vi "oa_Analog Tacho Hysteresis(1 Channel).vi"(0 "input signal":dbl[](array[numeric]), 1 "reset? (T)":bool=TRUE, 5 "threshold (auto)":dbl=inf format="%.2f", 7 "slope (Rising)":u16(ring) items=["Rising", "Falling"], 9 "hysteresis(0)":dbl format="%.2f", 11 "error in (no error)":errorcluster) -> (4 "output signal":dbl[](array[numeric]), 15 "error out":errorcluster)   [LabVIEW 2017, in "SoundVib_TachProcess.lvlib"]
doc: "This VI works like a hysteresis comparater. It can transform the input tachometer signal into a standard square waveform, ignoring small pulsed caused by harmonics or noise. By setting the hystersis value properly, it can make the speed tracking more accurately."
uses:
  <vilib>/addons/Sound and Vibration/Order Analysis/Tach Process/SoundVib_TachProcess.lvlib
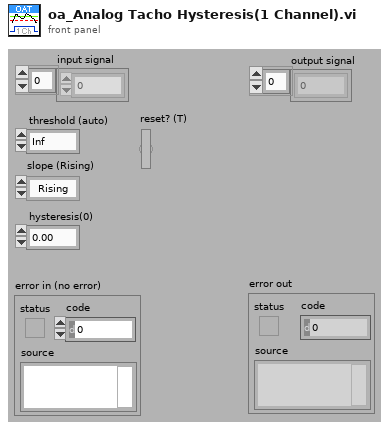
[diagram p1: front panel]
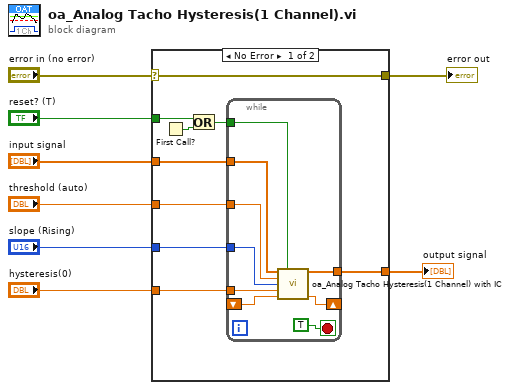
[diagram p0: block diagram]
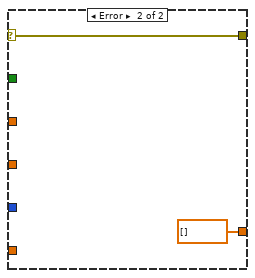
[diagram p2: hidden frame]
diagram:
  n1 = case shown="No Error" "error in (no error)" {
    selector: "error in (no error)" -> [w15 w28]
    tunnel: "reset? (T)" -> [w16 _]
    tunnel: "hysteresis(0)" -> [w10 _]
    tunnel: "threshold (auto)" -> [w11 _]
    tunnel: "slope (Rising)" -> [w13 _]
    tunnel: [w9 dbl[] [] ("signal")] -> w1
    tunnel: [w15 w28] -> w3
    tunnel: "input signal" -> [w12 _]
    frame No Error {
      n2 = First Call?() -> (First Call?: T/F=w17:bool)
      n3 = Or(x=w16, y=w17) -> (x .or. y?=w14:bool)
      n4 = while {
        tunnel: w14 -> [w26]
        tunnel: w13 -> [w25]
        tunnel: w12 -> [w24]
        tunnel: w11 -> [w23]
        tunnel: w10 -> [w22]
        shift-right: [w21] -> _
        shift-left: _ -> [w20]
        tunnel: [w19] -> w9
        stop <- TRUE stop-if-true
        n5 = call <vilib>:"oa_Analog Tacho Hysteresis(1 Channel) with IC.vi"("input signal"=w24, "reset? (T)"=w26, "threshold (auto)"=w23, "slope (Rising)"=w25, "hysteresis(0)"=w22, "initial condition"=w20) -> ("output signal"=w19:dbl[], "final condition"=w21:dbl)  [unwired: 8 in]
      }
    }
    frame Error {
    }
  }
  "error out" <- w3
  "output signal" <- w1
